vi "myRIO_BRig_RT_dataExp_CueLed_Freq.vi"() -> (2 "output_CueLed_Freq":i32)   [LabVIEW 2014]
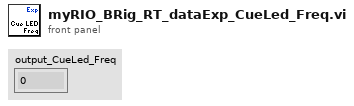
[diagram p1: front panel]
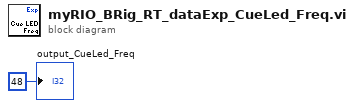
[diagram p0: block diagram]
diagram:
  "output_CueLed_Freq" <- 48 ("output_iBlock")
